vi "Initial Password.vi"(8 "error in (no error)":errorcluster, 11 "Master in":refnum<class "MASTER.lvclass">) -> (0 "error out":errorcluster, 3 "Master out":refnum<class "MASTER.lvclass">)   [LabVIEW 2014, in "Files Library.lvlib" / "Master.lvclass"]
uses:
  MASTER/MASTER.lvclass
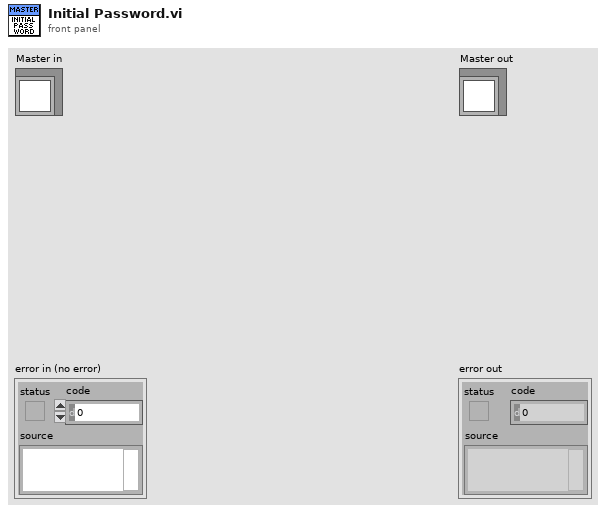
[diagram p1: front panel]
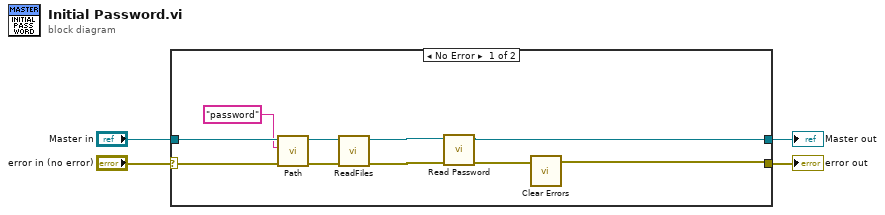
[diagram p0: block diagram]
diagram:
  n1 = case shown="No Error" "error in (no error)" {
    selector: "error in (no error)" -> [w12 w16]
    tunnel: [w6 w16] -> w3
    tunnel: [w5 w15] -> w1
    tunnel: "Master in" -> [w14 w15]
    frame No Error {
      n2 = call-dynamic "Path.vi"("error in (no error)"=w12, "pathname"="password", "Master in"=w14) -> ("error out"=w11:errorcluster, "Master out"=w13:refnum<class "MASTER.lvclass">)  [unwired: 7 in]
      n3 = call-dynamic "ReadFiles.vi"("error in (no error)"=w11, "Master in"=w13) -> ("error out"=w8:errorcluster, "Master out"=w9:refnum<class "MASTER.lvclass">)  [unwired: 8 in]
      n4 = call-dynamic "Read Password.vi"("error in (no error)"=w8, "Master in"=w9) -> ("error out"=w7:errorcluster, "Master out"=w5:refnum<class "MASTER.lvclass">)  [unwired: 8 in]
      n5 = call <vilib>:"Clear Errors.vi"("error in (no error)"=w7) -> ("error out"=w6:errorcluster)  [unwired: 5 in, 1 out]
    }
    frame Error {
    }
  }
  "error out" <- w3
  "Master out" <- w1
